vi "MultiplyMatrixElements.vi"(1 "Element2":string, 2 "Element1":string) -> (0 "Element Out":string)   [LabVIEW 2011]
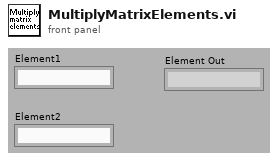
[diagram p1: front panel]
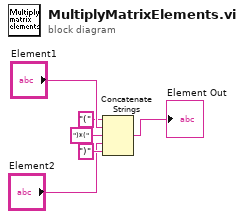
[diagram p0: block diagram]
diagram:
  n1 = Concatenate Strings("(" ("string"), "Element1", ")*(" ("string"), "Element2", ")" ("string")) -> (→"Element Out":string)
